vi "Fft.vi"(10 "Chirp Parameters (in)":T1, 11 "DataPoints (in)":csg[](array[numeric])) -> (3 "Fft Results (out)":csg[](array[numeric]))   [LabVIEW 2015, in "SETI_LV.lvlib"]
uses:
  SETI_LV.lvlib
  TypeDefs/ChirpFFT Pairs.ctl
  <vilib>/Analysis/2dsp.llb/Complex FFT.vi
  <vilib>/Analysis/NI_AALPro.lvlib
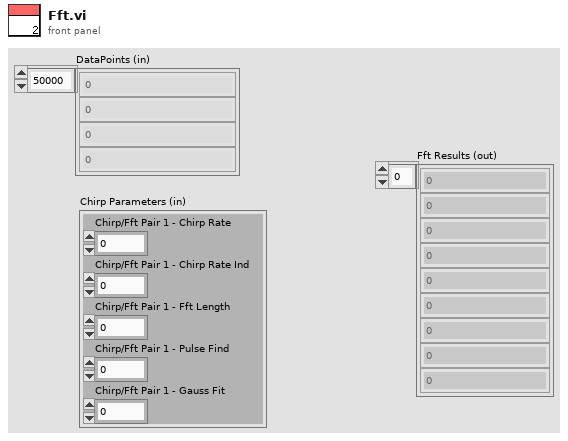
[diagram p1: front panel]
types:
  T1 = typedef "SETI_LV.lvlib/ChirpFFT Pairs.ctl" = cluster{"Chirp/Fft Pair 1 - Chirp Rate":dbl, "Chirp/Fft Pair 1 - Chirp Rate Ind":i32, "Chirp/Fft Pair 1 - Fft Length":i32, "Chirp/Fft Pair 1 - Pulse Find":i32, "Chirp/Fft Pair 1 - Gauss Fit":i32}
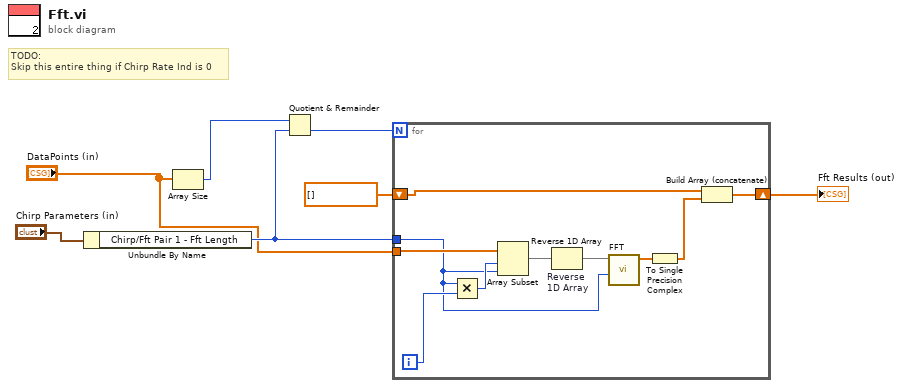
[diagram p0: block diagram]
diagram:
  # "TODO:\nSkip this entire thing if Chirp Rate Ind is 0"
  n1 = Unbundle By Name("Chirp Parameters (in)") -> ("Chirp/Fft Pair 1 - Fft Length"=w5:i32)
  n2 = Array Size(array="DataPoints (in)") -> (size(s)=w1:i32)
  n3 = Quotient & Remainder(x=w1, y=w5) -> (floor(x/y)=w6:i32)  [unwired: 1 out]
  n4 = for {
    N: w6 -> [_]
    tunnel: "DataPoints (in)" -> [w14]
    tunnel: w5 -> [w12]
    shift-right: [w11] -> w4
    shift-left: csg[] [] -> [w10]
    i -> [w13]
    n5 = Multiply(x=w12, y=w13) -> (x*y=w17:i32)
    n6 = Array Subset(array=w14, index=w17, length=w12) -> (w16:csg[])
    n7 = Reverse 1D Array "Reverse\n1D Array"(array=w16) -> (reversed array=w15:csg[])
    n8 = call-poly <vilib>:"FFT.vi"("FFT size"=w12, "X"=w15) -> ("FFT {X}"=w9:cdb[])  [unwired: 8 in, 1 out]
    n9 = To Single Precision Complex(1:w9) -> (0:w8:csg[])
    n10 = Build Array (concatenate)(w10, w8) -> (w11:csg[])
  }
  "Fft Results (out)" <- w4
